vi "Write Accel & Gyro I2C.vi"(8 "error in (no error)":errorcluster, 10 "Accel/Gyro I2C":refnum<class "LINX I2C.lvclass">, 11 "LSM9DS1 in":refnum<class "LSM9DS1 IMU.lvclass">) -> (0 "error out":errorcluster, 3 "LSM9DS1 out":refnum<class "LSM9DS1 IMU.lvclass">)   [LabVIEW 2020, in "LSM9DS1 IMU.lvclass"]
uses:
  LSM9DS1 IMU.lvclass
  LINX I2C/LINX I2C.lvclass
  LSM9DS1 IMU.lvclass/LSM9DS1 IMU.ctl
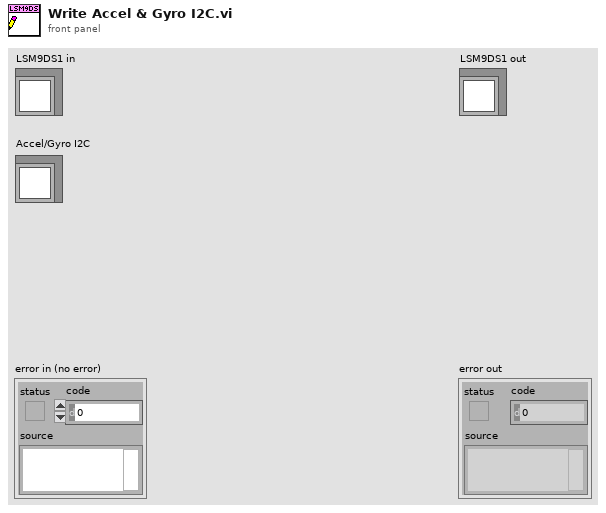
[diagram p1: front panel]
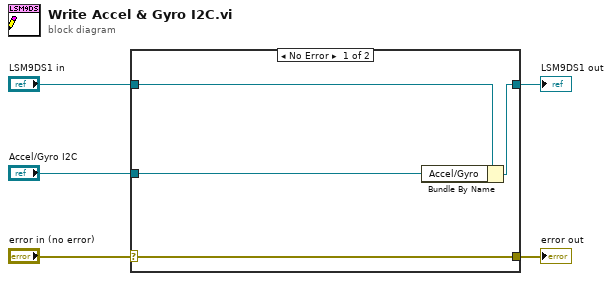
[diagram p0: block diagram]
diagram:
  n1 = case shown="No Error" "error in (no error)" {
    selector: "error in (no error)" -> [w9 w10]
    tunnel: [w9 w10] -> w4
    tunnel: [w7 w11] -> w2
    tunnel: "LSM9DS1 in" -> [w8 w11]
    tunnel: "Accel/Gyro I2C" -> [w6 _]
    frame No Error {
      n2 = Bundle By Name(cluster=w8, "Accel/Gyro"=w6) -> (w7:refnum<class "LSM9DS1 IMU.lvclass">)
    }
    frame Error {
    }
  }
  "error out" <- w4
  "LSM9DS1 out" <- w2
